vi "Move Steps.vi"(8 "error in (no error)":errorcluster, 10 "Number Of Steps":T1, 11 "Context in":refnum<class "Context.lvclass">) -> (0 "error out":errorcluster, 3 "Context out":refnum<class "Context.lvclass">)   [LabVIEW 2016, in "Context.lvclass"]
uses:
  Context.lvclass
  Typedefs/Number Of Steps.ctl
  Context.lvclass/Context.ctl
  States/State/State.lvclass
  Model/Model/Model.lvclass
  Typedefs/HPMT_Typedefs.lvlib
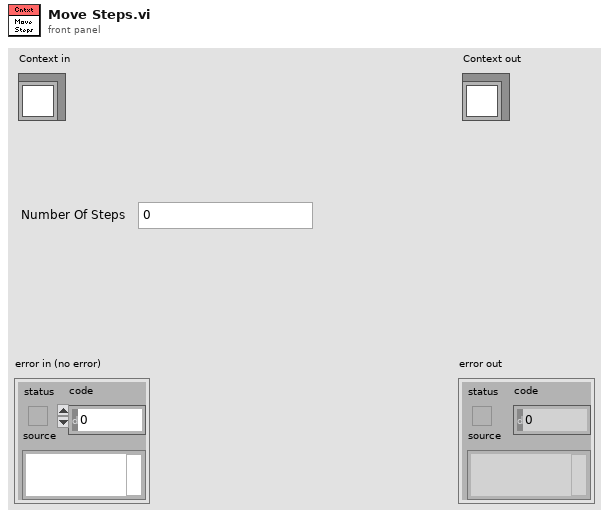
[diagram p1: front panel]
types:
  T1 = typedef "HPMT_Typedefs.lvlib/Number Of Steps.ctl" = i32
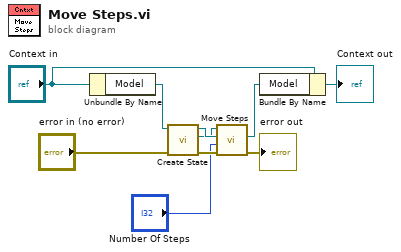
[diagram p0: block diagram]
diagram:
  n1 = Unbundle By Name("Context in") -> ("Model"=w8:refnum<class "Model.lvclass">)
  n2 = call "Create State.vi"("error in (no error)"="error in (no error)", "Model in"=w8) -> ("error out"=w3:errorcluster, "State"=w4:refnum<class "State.lvclass">, "Model out"=w6:refnum<class "Model.lvclass">)  [unwired: 7 in]
  n3 = call-dynamic "Move Steps.vi"("error in (no error)"=w3, "Number Of Steps"="Number Of Steps", "Model in"=w6, "State in"=w4) -> ("error out"=→"error out":errorcluster, "Model out"=w5:refnum<class "Model.lvclass">)  [unwired: 5 in, 1 out]
  n4 = Bundle By Name(cluster="Context in", "Model"=w5) -> (→"Context out":refnum<class "Context.lvclass">)
